vi "ToTab.vi"(8 "error in":errorcluster, 11 "Generic in":refnum<class "Generic.lvclass">) -> (0 "error out":errorcluster, 3 "Tab out":refnum<class "Tab.lvclass">)   [LabVIEW 2014, in "Tab.lvclass"]
uses:
  Tab.lvclass
  Generic/Generic.lvclass
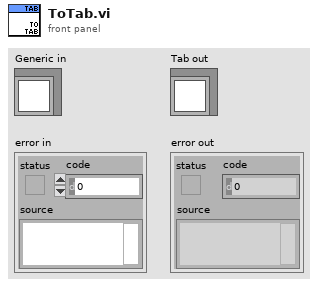
[diagram p1: front panel]
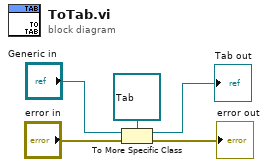
[diagram p0: block diagram]
diagram:
  n1 = To More Specific Class(target class=refnum<class "Tab.lvclass"> refnum ("Tab out"), reference="Generic in", error in="error in") -> (specific class reference=→"Tab out":refnum<class "Tab.lvclass">, error out=→"error out":errorcluster)
